vi "3.9 Mutation.vi"(8 "error in (no error)":errorcluster, 11 "Device Ref out":T1 format="%.0x") -> (0 "error out":errorcluster, 3 "Device Ref out":T1 format="%.0x")   [LabVIEW 2011, in "Engine Sim System Explorer.lvlib"]
uses:
  Engine Sim System Explorer.lvlib
  <vilib>/NI Veristand/Custom Device API/Custom Device Item Ref.ctl
  TypeDefs/DataReplayLoopComp.ctl
  TypeDefs/DataReplayComp.ctl
  Shared/Engine Simulation Global.vi
  <vilib>/NI Veristand/Custom Device Tools/Custom Device Utility Library/NI VeriStand - Search for Item by GUID.vi
  <vilib>/NI Veristand/Custom Device Tools/Custom Device Utility Library/NI VeriStand - Search for Item by Name.vi
  <vilib>/NI Veristand/Custom Device API/Get Item Property (Variant).vi
  <vilib>/NI Veristand/Custom Device Tools/Custom Device Utility Library/NI VeriStand - Search for All Items by GUID.vi
  <vilib>/NI Veristand/Custom Device Tools/Custom Device Utility Library/Custom Device Utility Library.lvlib
  Engine Simulation Shared.lvlib
  <vilib>/NI Veristand/Custom Device API/Custom Device API.lvlib
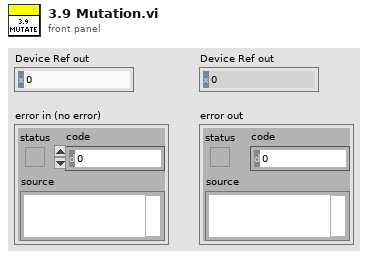
[diagram p1: front panel]
types:
  T1 = typedef "Custom Device API.lvlib/Custom Device Item Ref.ctl" = u64
  T2 = cluster{"Name":string, "DataReplays":cluster{"Name":string, "Number":i8}[]}[]
  T3 = typedef "Engine Sim System Explorer.lvlib/DataReplayLoopComp.ctl" = cluster{"Name":string, "DataReplays":T4[]}
  T4 = typedef "Engine Sim System Explorer.lvlib/DataReplayComp.ctl" = cluster{"Name":string, "Number":i32, "Optionals":bool[]}
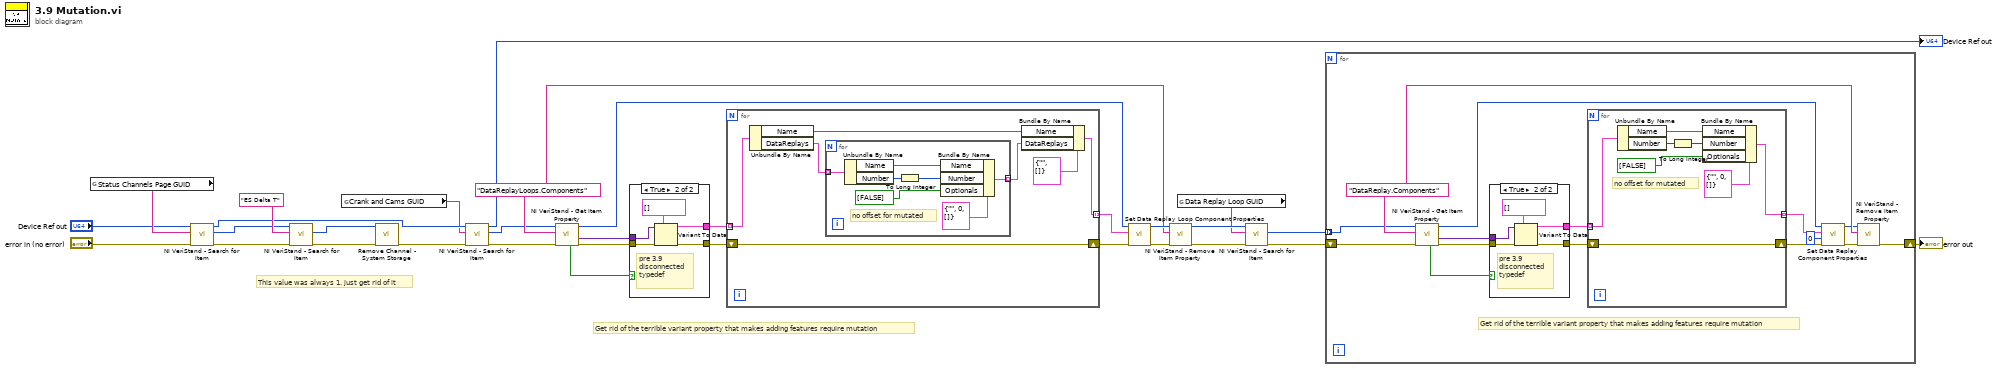
[diagram p0: block diagram]
diagram:
  w9 = "DataReplayLoops.Components" ("Item GUID")
  # "Get rid of the terrible variant property that makes adding features require mutation"
  # "This value was always 1. just get rid of it"
  n1 = global read "Engine Simulation Global.vi" "Status Channels Page GUID"() -> (w25:string)
  n2 = call-poly <vilib>:"NI VeriStand - Search for Item.vi"("error in"="error in (no error)", "Item GUID"=w25, "Section Ref in"="Device Ref out") -> ("error out"=w28:errorcluster, "Item Ref"=w26:T1, "Section Ref out"=w21:T1)  [unwired: 5 in, 1 out]
  n3 = call-poly <vilib>:"NI VeriStand - Search for Item.vi"("error in"=w28, "Item Name"="ES Delta T" ("Item GUID"), "Section Ref in"=w26) -> ("error out"=w29:errorcluster, "Item Ref"=w31:T1)  [unwired: 5 in, 2 out]
  n4 = global read "Engine Simulation Global.vi" "Crank and Cams GUID"() -> (w20:string)
  n5 = call "Remove Channel - System Storage.vi"("error in (no error)"=w29, "Channel ref in"=w31) -> ("error out"=w30:errorcluster)  [unwired: 9 in]
  n6 = call-poly <vilib>:"NI VeriStand - Search for Item.vi"("error in"=w30, "Item GUID"=w20, "Section Ref in"=w21) -> ("error out"=w22:errorcluster, "Item Ref"=w8:T1, "Section Ref out"=→"Device Ref out":T1)  [unwired: 5 in, 1 out]
  n7 = call-poly <vilib>:"NI VeriStand - Get Item Property.vi"("error in (no error)"=w22, "Property Name"=w9, "Item Ref in"=w8) -> ("error out"=w18:errorcluster, "Value"=w17:variant, "Item Ref out"=w14:T1, "Found?"=w19:bool)  [unwired: 5 in]
  n8 = case shown="True" w19 {
    tunnel: w18 -> [w32 w37]
    tunnel: w17 -> [_ w36]
    tunnel: [w32 w35] -> w13
    tunnel: [_ w34] -> w16
    frame False {
    }
    frame True {
      # "pre 3.9 disconnected typedef"
      n9 = Variant To Data(error in=w37, type=T2 [], Variant=w36) -> (data=w34:T2, error out=w35:errorcluster)
    }
  }
  n10 = for {
    tunnel: w16 -> [w43] mode=indexing
    tunnel: [w41] -> w15 mode=indexing
    shift-right: [w39] -> w12
    shift-left: w13 -> [w39]
    n11 = Unbundle By Name(w43) -> ("Name"=w42:string, "DataReplays"=w40:cluster{"Name":string, "Number":i8}[])
    n12 = for {
      tunnel: w40 -> [w51] mode=indexing
      tunnel: [w45] -> w38 mode=indexing
      # "no offset for mutated"
      n13 = Unbundle By Name(w51) -> ("Name"=w49:string, "Number"=w48:i8)
      n14 = To Long Integer(number=w48) -> (32bit integer=w47:i32)
      n15 = Bundle By Name(cluster=T4 {"Name"="", "Number"=0, "Optionals"=[]} ("DataReplay"), "Name"=w49, "Number"=w47, "Optionals"=bool[] [FALSE]) -> (w45:T4)
    }
    n16 = Bundle By Name(cluster=T3 {"Name"="", "DataReplays"=[]} ("DataReplayLoop"), "Name"=w42, "DataReplays"=w38) -> (w41:T3)
  }
  n17 = call "Set Data Replay Loop Component Properties.vi"("error in (no error)"=w12, "DataReplayLoops"=w15, "Item Ref in"=w14) -> ("error out"=w11:errorcluster, "Item Ref out"=w10:T1)  [unwired: 7 in]
  n18 = call <vilib>:"NI VeriStand - Remove Item Property.vi"("error in (no error)"=w11, "Property Name"=w9, "Item Ref in"=w10) -> ("error out"=w7:errorcluster, "Item Ref out"=w6:T1)  [unwired: 6 in, 1 out]
  n19 = global read "Engine Simulation Global.vi" "Data Replay Loop GUID"() -> (w5:string)
  n20 = call-poly <vilib>:"NI VeriStand - Search for Item.vi"("error in"=w7, "Item GUID"=w5, "Section Ref in"=w6) -> ("error out"=w4:errorcluster, "Item Refs"=w3:T1[])  [unwired: 5 in, 2 out]
  n21 = for {
    shift-right: [w52] -> w2
    shift-left: w4 -> [w56]
    tunnel: w3 -> [w55] mode=indexing
    w66 = "DataReplay.Components" ("Item GUID")
    # "Get rid of the terrible variant property that makes adding features require mutation"
    n22 = call-poly <vilib>:"NI VeriStand - Get Item Property.vi"("error in (no error)"=w56, "Property Name"=w66, "Item Ref in"=w55) -> ("error out"=w58:errorcluster, "Value"=w59:variant, "Item Ref out"=w61:T1, "Found?"=w57:bool)  [unwired: 5 in]
    n23 = case shown="True" w57 {
      tunnel: w58 -> [w75 w80]
      tunnel: w59 -> [_ w79]
      tunnel: [w75 w78] -> w62
      tunnel: [_ w77] -> w60
      frame False {
      }
      frame True {
        # "pre 3.9 disconnected typedef"
        n24 = Variant To Data(error in=w80, type=cluster{"Name":string, "Number":i8}[] [], Variant=w79) -> (data=w77:cluster{"Name":string, "Number":i8}[], error out=w78:errorcluster)
      }
    }
    n25 = for {
      tunnel: w60 -> [w74] mode=indexing
      tunnel: [w67] -> w54 mode=indexing
      shift-right: [w73] -> w63
      shift-left: w62 -> [w73]
      # "no offset for mutated"
      n26 = Unbundle By Name(w74) -> ("Name"=w70:string, "Number"=w69:i8)
      n27 = To Long Integer(number=w69) -> (32bit integer=w68:i32)
      n28 = Bundle By Name(cluster=T4 {"Name"="", "Number"=0, "Optionals"=[]} ("DataReplay"), "Name"=w70, "Number"=w68, "Optionals"=bool[] [FALSE]) -> (w67:T4)
    }
    n29 = call "Set Data Replay Component Properties.vi"("error in (no error)"=w63, "Prefix#"=0, "DataReplays"=w54, "Item Ref in"=w61) -> ("error out"=w64:errorcluster, "Item Ref out"=w65:T1)  [unwired: 6 in]
    n30 = call <vilib>:"NI VeriStand - Remove Item Property.vi"("error in (no error)"=w64, "Property Name"=w66, "Item Ref in"=w65) -> ("error out"=w52:errorcluster)  [unwired: 6 in, 2 out]
  }
  "error out" <- w2
